vi "Power_Supply_GUI.vi"(8 "error in (no error)":errorcluster, 11 "Instrument Reference":u8) -> (0 "error out":errorcluster)   [LabVIEW 2018, in "PXIe-4130.lvclass"]
uses:
  PXIe-4130.lvclass
  Power_Supply Virtual/Power_Supply Virtual.lvclass
panel:
  out "Sub Address":string
  out "Model Number":string
  in  "stop":bool
  # "PXIe-4130 GUI"
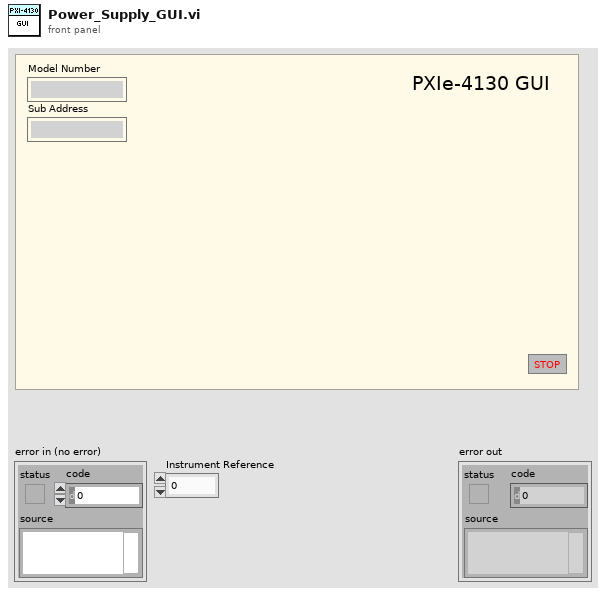
[diagram p1: front panel]
types:
  T1 = typedef "Class Attributes Cluster.ctl" = cluster{"Model Number":string, "Instrument Number":u8, "Rack ID":string, "Inst Mnemonic":string, "Comp Mnemonic":string, "Subsys Mnemonic":string, "IP Address":string, "Sub Address":string, "Firmware Rev":string, "Expected Options":string, "Required Options":string, "Excluded Options":string}
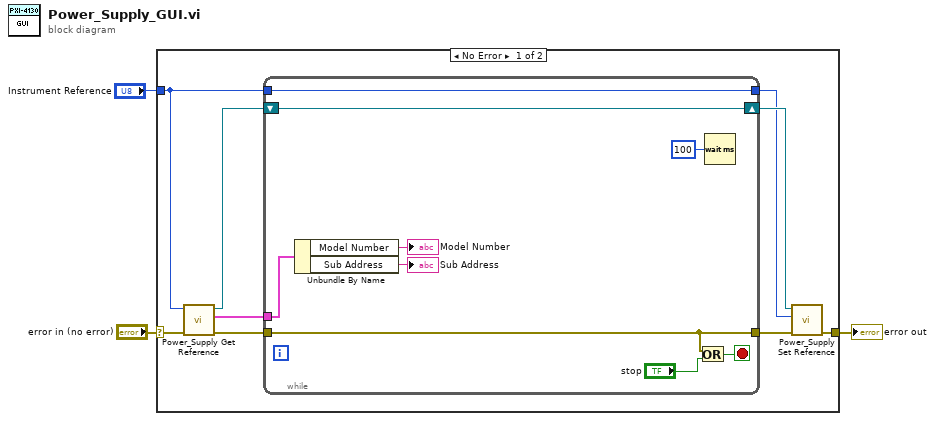
[diagram p0: block diagram]
diagram:
  n1 = case shown="No Error" "error in (no error)" {
    selector: "error in (no error)" -> [w12 w22]
    tunnel: [w7 w22] -> w1
    tunnel: "Instrument Reference" -> [w5 _]
    frame No Error {
      n2 = call "Power_Supply Get Reference.vi"("error in (no error)"=w12, "Instrument Reference"=w5) -> ("error out"=w11:errorcluster, "Class Attributes"=w9:T1, "Power_Supply Virtual.lvclass"=w10:refnum<class "Power_Supply Virtual.lvclass">)  [unwired: 7 in]
      n3 = while {
        tunnel: w11 -> [w20]
        tunnel: [w20] -> w8
        shift-right: [w21] -> w6
        shift-left: w10 -> [w21]
        tunnel: w9 -> [w14]
        tunnel: w5 -> [w13]
        tunnel: [w13] -> w4
        stop <- w18 stop-if-true
        n4 = Unbundle By Name(w14) -> ("Model Number"=→"Model Number":string, "Sub Address"=→"Sub Address":string)
        n5 = Or(x=w20, y="stop") -> (x .or. y?=w18:bool)
        n6 = Wait (ms)(milliseconds to wait=u32 100) -> ()  [unwired: 1 out]
      }
      n7 = call "Power_Supply Set Reference.vi"("error in (no error)"=w8, "User Reference"=w4, "Power_Supply Virtual.lvclass"=w6) -> ("error out"=w7:errorcluster)  [unwired: 8 in]
    }
    frame Error {
    }
  }
  "error out" <- w1
